vi "Agilent 2000 3000 X-Series Frequency Response Analysis.vi"() -> ()   [LabVIEW 2015]
doc: "This example shows how to configure frequency response analysis and read the measurement data. \n\n<b>Notes:</b>:\nThis example is only applicable for 1000 Series."
uses:
  Agilent 2000 3000 X-Series.lvlib
panel:
  in  "Start Frequency (0: 20Hz)":i32(ring) items=["20Hz", "100Hz", "1KHz", "10KHz", "100KHz", "1MHz", "10MHz", "10Hz", "20MHz"]
  in  "Stop Frequency (0: 100Hz)":i32(ring) items=["100Hz", "1KHz", "10KHz", "100KHz", "1MHz", "10MHz", "20MHz"]
  in  "Load Resistance (0: 1 Mohm)":i32(ring) items=["1 Mohm", "50 ohm"]
  in  "Output Source (1: Channel 2)":i32(ring)=1 items=["Channel 1", "Channel 2", "Channel 3", "Channel 4"]
  in  "Input Voltage Amplitude (1 Volts)":dbl=1.0
  in  "Input Source (0: Channel 1)":i32(ring) items=["Channel 1", "Channel 2", "Channel 3", "Channel 4"]
  in  "VISA resource name":refnum<visa-resource-name>
  out "Frequency Analysis Data":dbl[][](array[numeric])
  # "(c) 2011-2023 National Instruments.  ALL RIGHTS RESERVED."
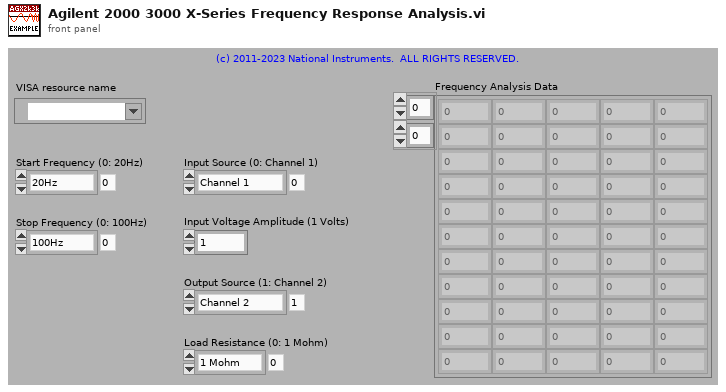
[diagram p1: front panel]
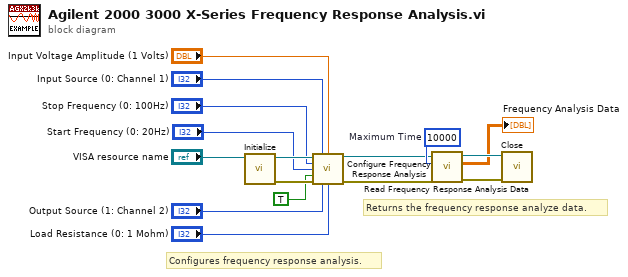
[diagram p0: block diagram]
diagram:
  w5 = u32 10000  # Maximum Time
  # "Returns the frequency response analyze data."
  # "Configures frequency response analysis."
  n1 = call "Initialize.vi"("VISA resource name"="VISA resource name") -> ("error out"=w14:errorcluster, "VISA resource name out"=w16:refnum<visa-resource-name>)  [unwired: 9 in]
  n2 = call "Configure Frequency Response Analysis.vi"("VISA resource name"=w16, "Input Source (0: Channel 1)"="Input Source (0: Channel 1)", "Input Voltage Amplitude (1 Volts)"="Input Voltage Amplitude (1 Volts)", "Stop Frequency (0: 100Hz)"="Stop Frequency (0: 100Hz)", "Start Frequency (0: 20Hz)"="Start Frequency (0: 20Hz)", "Enable Frequency Response Analysis (F: Disable)"=TRUE, "error in (no error)"=w14, "Output Source (1: Channel 2)"="Output Source (1: Channel 2)", "Load Resistance (0: 1 Mohm)"="Load Resistance (0: 1 Mohm)") -> ("VISA resource name out"=w4:refnum<visa-resource-name>, "error out"=w3:errorcluster)  [unwired: 5 in]
  n3 = call "Read Frequency Response Analysis Data.vi"("error in (no error)"=w3, "Maximum Time (10000)"=w5, "VISA resource name"=w4) -> ("error out"=w13:errorcluster, "Frequency Analysis Data"=→"Frequency Analysis Data":dbl[][], "VISA resource name out"=w15:refnum<visa-resource-name>)  [unwired: 6 in]
  n4 = call "Close.vi"("error in (no error)"=w13, "VISA resource name"=w15) -> ()  [unwired: 9 in, 1 out]
